vi "find nearest voltage range.vi"(11 "Range in":dbl) -> (3 "Range":u16(ring)=6 items=["10 mV", "20 mV", "50 mV", "100 mV", "200 mV", "500 mV", "1 V", "2 V", "5 V", "10 V", "20 V", "50 V ", "100 V"])   [LabVIEW 2020]
uses:
  LVStringsAndValuesArrayTypeDef_U16.ctl
panel:
  out "nearest Range":dbl
  out "Array 2":string[](array[string])
  out "Voltage ranges":dbl[](array[numeric])
  out "Strings And Values []":T1
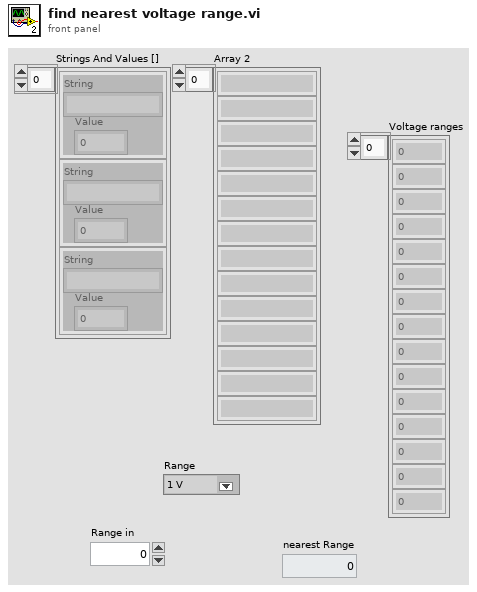
[diagram p1: front panel]
types:
  T1 = typedef "LVStringsAndValuesArrayTypeDef_U16.ctl" = cluster{"String":string, "Value":u16}[]
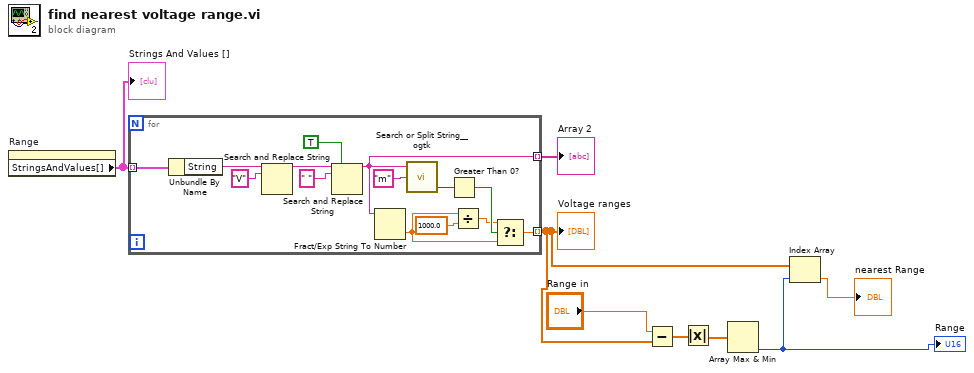
[diagram p0: block diagram]
diagram:
  n1 = property on="Range" class="Ring (strict)"() -> ("StringsAndValues[]"=w8:T1)  [unwired: 2 in, 2 out]
  "Strings And Values []" <- w8
  n2 = for {
    tunnel: w8 -> [w22] mode=indexing
    tunnel: [w13] -> w3 mode=indexing
    tunnel: [w16] -> w7 mode=indexing
    n3 = Unbundle By Name(w22) -> ("String"=w21:string)
    n4 = Search and Replace String(input string=w21, search string="V") -> (result string=w18:string)  [unwired: 6 in, 3 out]
    n5 = Search and Replace String(replace all?=TRUE ("replace all? (F)"), input string=w18, search string=" ") -> (result string=w16:string)  [unwired: 5 in, 3 out]
    n6 = Fract/Exp String To Number(string=w16) -> (number=w12:dbl)  [unwired: 3 in, 1 out]
    n7 = call "Search or Split String__ogtk.vi"("search string/char (-)"="m", "string"=w16) -> ("offset after match"=w14:i32)  [unwired: 1 in, 2 out]
    n8 = Greater Than 0?(x=w14) -> (x > 0?=w11:bool)
    n9 = Divide(x=w12, y=1000.0) -> (x/y=w9:dbl)
    n10 = Select(t=w9, s=w11, f=w12) -> (s? t:f=w13:dbl)
  }
  "Voltage ranges" <- w3
  "Array 2" <- w7
  n11 = Subtract(x="Range in", y=w3) -> (x-y=w5:dbl[])
  n12 = Absolute Value(x=w5) -> (abs(x)=w4:dbl[])
  n13 = Array Max & Min(array=w4) -> (min index (indices)=w1:i32)  [unwired: 3 out]
  "Range" <- w1
  n14 = Index Array(array=w3, index=w1) -> (element=→"nearest Range":dbl)
